vi "Demultiplexer_Laser80VerySimple160.vi"() -> ()   [LabVIEW 2012]
uses:
  <vilib>/Platform/TimedLoop/XDataNode/timing_clust.ctl
  <vilib>/Platform/TimedLoop/XDataNode/nitl_modes.ctl
  <vilib>/Platform/TimedLoop/XDataNode/wakeup.ctl
  <vilib>/rvi/Emulation/niFpgaSctlEmulationRegisterWithScheduler.vi
  <vilib>/rvi/eio/common/nirviEmuTemplateMethod_errors.vi
  <vilib>/rvi/Emulation/niFpgaSctlEmulationScheduler.vi
  <vilib>/rvi/FIFO/Fifo_Resource/nirvififoEmulationSetSize.vi
  <vilib>/rvi/DataTransferAndStorage/Container/Common/niFpgaContainerGetUniqueNameForEmu.vi
  <vilib>/rvi/errors/niFpgaSetErrorForExecOnDevCompSimple.vi
  <vilib>/rvi/eio/common/nirviEmuReportErrorAndStop.vi
  <vilib>/rvi/Emulation/niFpgaSctlEmulationFifoFullMgr.vi
  <vilib>/rvi/Emulation/niFpgaSctlEmulationResourceMgr.vi
  <vilib>/rvi/interface/RandomDataEmulation/nirviRandomDataFPGAFIFO.vi
  <vilib>/rvi/interface/RandomDataEmulation/niFpgaRandomDataHandleErrors.vi
  <vilib>/rvi/Emulation/niFpgaSctlEmulationGlobalWrite.vi
  <vilib>/Platform/TimedLoop/XDataNode/XDataNode.xnode
  <vilib>/eio/EIONode/EIONode.xnode
  <vilib>/rvi/DataTransferAndStorage/Container/XNode/niFpgaContainer.xnode
  <vilib>/rvi/FIFO/Fifo_Resource/nirvififoEmulationClear.vi
  <vilib>/rvi/FIFO/Fifo_Resource/nirvififoEmulationWrite.vi
  <vilib>/rvi/FIFO/Fifo_Resource/nirvififoEmulationRead.vi
  <vilib>/rvi/interface/RandomDataEmulation/nirviRandomDataFpgaReadWriteTemplate.vi
  <vilib>/Platform/TimedLoop/XDataNode/XDNodeRunTimeDep.lvlib
panel:
  out "Laser pulses per pixel A1":u16
  out "ToHost FIFO Overflow A2Ch2":bool
  out "ToHost FIFO Overflow A2Ch1":bool
  out "ToHost FIFO Overflow A1Ch2":bool
  in  "Samples per pixel Acq A2":u16=10000 caption="Samples per pixel Acq"
  in  "Samples per pixel Acq A1":u16=10000 caption="Samples per pixel Acq"
  in  "Requested pixels A2":u32=100000 caption="Requested pixels"
  in  "Samples per pixel A2":u16=10000 caption="Samples per pixel"
  out "ToHost FIFO Overflow A1Ch1":bool
  out "Acquiring":bool
  in  "Wait for trigger":bool
  in  "Acquire continuously":bool=TRUE
  in  "Requested pixels A1":u32=100000 caption="Requested pixels"
  in  "Clear Interloop FIFO":bool
  out "Interloop FIFO overflow":bool
  in  "Samples per pixel A1":u16=10000 caption="Samples per pixel"
  in  "Acquire":bool
  out "Interloop FIFO timeout":bool
  in  "Commit":bool
  out "Xpoint_Switch_Ready":bool
  in  "Xpoint_Switch_Write":bool
  in  "Clock Source":u8(ring)=3 items=["Tristate"=0, "Sync Clock (PXIe only)"=2, "Adapter Module Onboard Clock"=3, "Strobe from Crosspoint Switch"=4, "Strobe Bypass"=5]
  in  "Onboard_Clock_Write":bool
  in  "Onboard_Clock_Write_Data":u16
  out "Onboard_Clock_Ready":bool
  in  "Acq_Reset":bool
  # "6587 IO module configuration"
  # "Demultiplexer - Laser 80MHzVerySimple160MHz"
  # "Acquisition control"
  # "Area 1"
  # "Area 2"
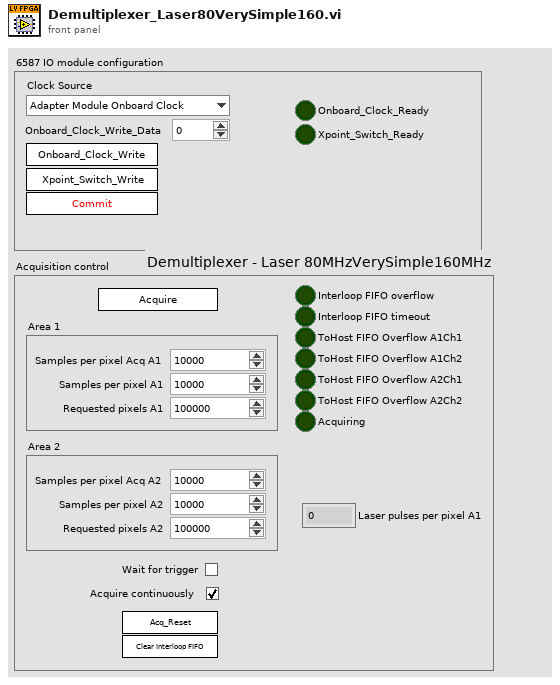
[diagram p1: front panel]
types:
  T1 = typedef "XDNodeRunTimeDep.lvlib/timing_clust.ctl" = cluster{"Expected End [f-1]":u64, "Actual End [f-1]":u64, "Finished Late? [f-1]":bool, "Expected End [i-1]":u64, "Actual End [i-1]":u64, "Finished Late? [i-1]":bool, "Expected Start [i]":u64, "Actual Start [i]":u64, "Expected Start [f]":u64, "Actual Start [f]":u64, "Source Name":string, "Structure Name":string, "Period":i64, "Deadline":i64, "Offset":i64, "Start":i64, "Priority":i32, "Timeout":i32, "Mode":T2, "Wakeup Reason":T3, "Error":errorcluster, "Source Type":string, "Secondary Source Type":string, "Global End Time":u64, "Global Start Time":u64, "Frame Duration":u64, "Iteration Duration":u64, "Assigned CPU":i32, "I/O Scan Engine Mode":u32}
  T2 = typedef "XDNodeRunTimeDep.lvlib/nitl_modes.ctl" = enum32{"No Change", "Process missed periods, maintain original phase", "Discard missed periods, maintain original phase", "Process missed periods, ignore original phase", "Discard missed periods, ignore original phase"}
  T3 = typedef "XDNodeRunTimeDep.lvlib/wakeup.ctl" = enum32{"Normal", "Aborted", "Asynchronous wakeup", "Timing source error", "Timed loop error", "Timeout"}
  T4 = cluster{"Laser":u64, "A1Ch1":u64, "A1Ch2":u64, "A2Ch1":u64, "A2Ch2":u64}
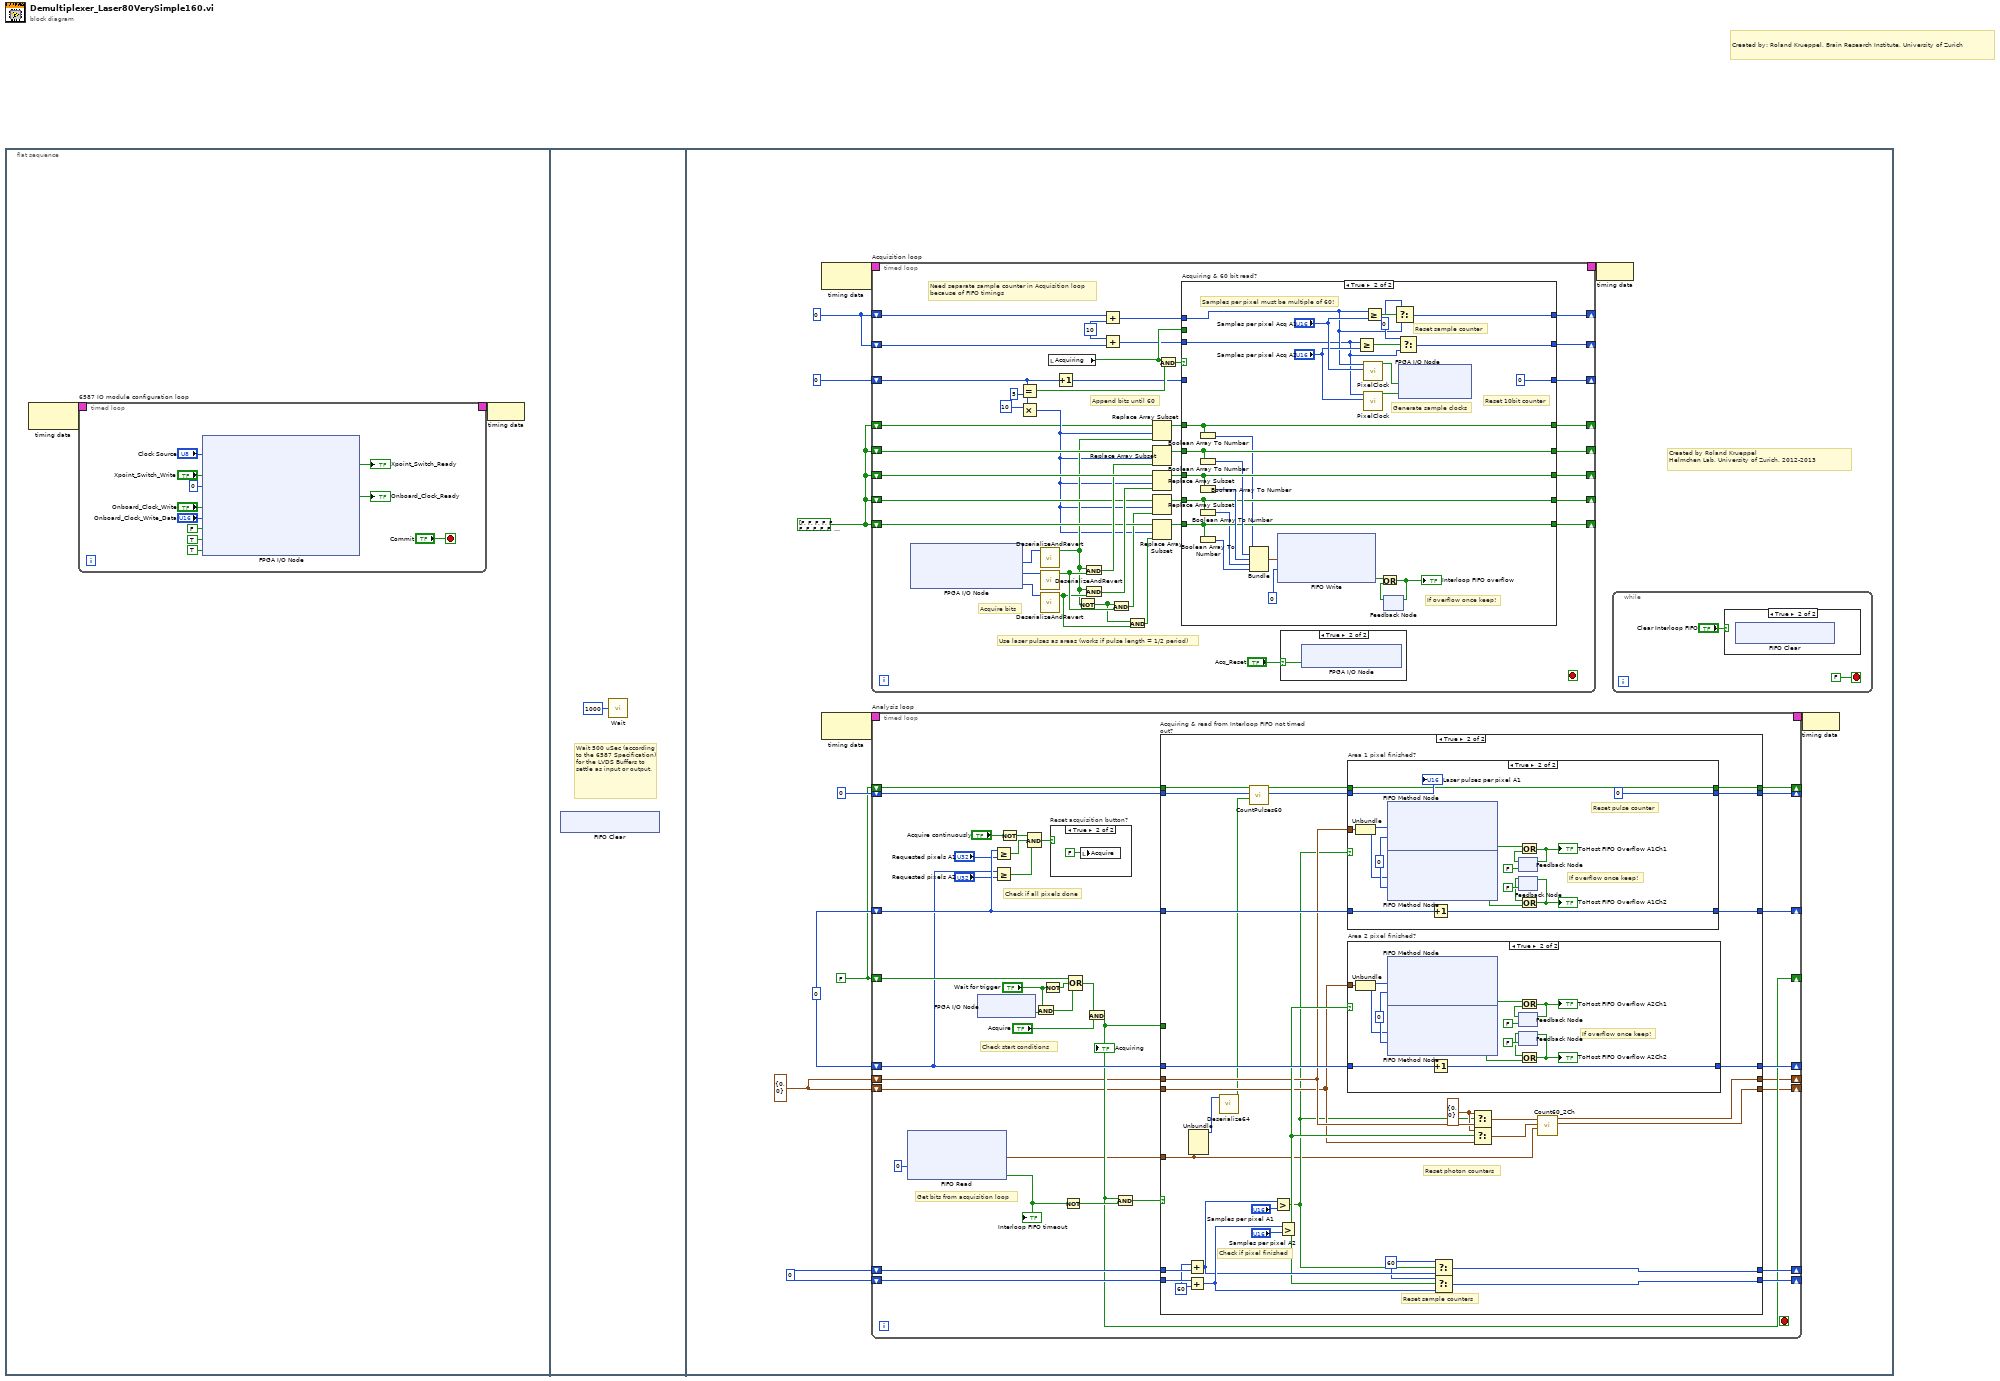
[diagram p0: block diagram]
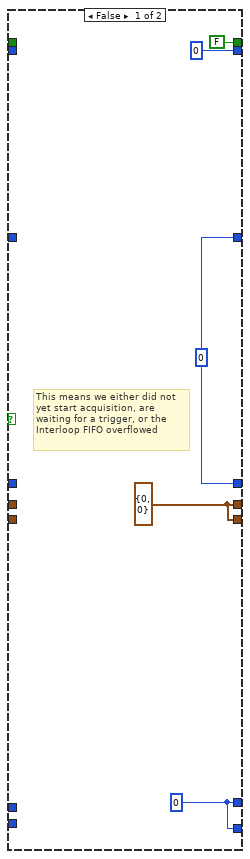
[diagram p5: hidden frame]
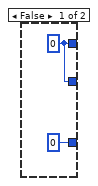
[diagram p10: hidden frame]
diagram:
  # "Created by: Roland Krueppel, Brain Research Institute, University of Zurich"
  n1 = flat-sequence {
    frame #0 {
      n2 = node-c288() -> (w2:T1)  [unwired: 1 in]
      n3 = timed-loop "6587 IO module configuration loop" {
        timing: w2 -> [_]
        timing-out: [_] -> w1
        stop <- "Commit" stop-if-true
        n4 = xnode "FPGA I/O Node"("IO Module\\Acq_IO_Clock_Source"="Clock Source", "IO Module\\Xpoint_Switch_Write"="Xpoint_Switch_Write", "IO Module\\LVDS_Data_Dir"=u16 0 ("IO Module\\LVDS_Data_Dir"), "IO Module\\Onboard_Clock_Write"="Onboard_Clock_Write", "IO Module\\Onboard_Clock_Write_Data"="Onboard_Clock_Write_Data", "IO Module\\SE_PFI0_WE"=FALSE ("IO Module\\SE_PFI0_WE"), "IO Module\\SE_PFI1_WE"=TRUE ("IO Module\\SE_PFI1_WE"), "IO Module\\SE_PFI2_WE"=TRUE ("IO Module\\SE_PFI2_WE")) -> ("IO Module\\Xpoint_Switch_Ready"=→"Xpoint_Switch_Ready":bool, "IO Module\\Onboard_Clock_Ready"=→"Onboard_Clock_Ready":bool)  [unwired: 10 in, 10 out]
      }
      n5 = node-c288(w1) -> ()
    }
    frame #1 {
      # "Wait 500 uSec (according to the 6587 Specification) for the LVDS Buffers to settle as input or output."
      n6 = xnode ("FIFO Clear")() -> ()  [unwired: 1 in, 1 out]
      n7 = call "Wait"("Count(uSec)"=u32 1000) -> ()  [unwired: 1 out]
    }
    frame #2 {
      w23 = cluster{u16, u16} {0, 0} ("output cluster")
      w24 = u16 0
      w22 = u32 0 ("Cycle counter out")
      w25 = u16 0
      w21 = bool[] [FALSE, FALSE, FALSE, FALSE, FALSE, FALSE, FALSE, FALSE, FALSE, FALSE, FALSE, FALSE, FALSE, FALSE, FALSE, FALSE, FALSE, FALSE, FALSE, FALSE, FALSE, FALSE, FALSE, FALSE, FALSE, FALSE, FALSE, FALSE, FALSE, FALSE, FALSE, FALSE, FALSE, FALSE, FALSE, FALSE, FALSE, FALSE, FALSE, FALSE, FALSE, FALSE, FALSE, FALSE, FALSE, FALSE, FALSE, FALSE, FALSE, FALSE, FALSE, FALSE, FALSE, FALSE, FALSE, FALSE, FALSE, FALSE, FALSE, FALSE, FALSE, FALSE, FALSE, FALSE] ("Boolean array")
      w19 = FALSE ("Last laser bit out")
      # "Created by Roland Krueppel\nHelmchen Lab, University of Zurich, 2012-2013"
      n8 = node-c288() -> (w30:T1)  [unwired: 1 in]
      n9 = node-c288() -> (w28:T1)  [unwired: 1 in]
      n10 = timed-loop "Acquisition loop" {
        timing: w30 -> [_]
        timing-out: [_] -> w29
        shift-right: [w207] -> _
        shift-left: w21 -> [w213]
        shift-right: [w206] -> _
        shift-left: 0 -> [w205]
        shift-right: [w202] -> _
        shift-left: w21 -> [w204]
        shift-right: [w201] -> _
        shift-left: w24 -> [w194]
        shift-right: [w200] -> _
        shift-left: w24 -> [w192]
        shift-right: [w177] -> _
        shift-left: w21 -> [w186]
        shift-right: [w176] -> _
        shift-left: w21 -> [w185]
        shift-right: [w171] -> _
        shift-left: w21 -> [w173]
        stop <- _ stop-if-true
        w190 = u16 10 ("y")
        # "Use laser pulses as areas (works if pulse length = 1/2 period)"
        # "Need separate sample counter in Acquisition loop\nbecause of FIFO timings"
        # "Append bits until 60"
        # "Acquire bits"
        n11 = xnode "FPGA I/O Node"() -> ("IO Module\\LVDS_Ch0_Rd"=w197:u16, "IO Module\\LVDS_Ch1_Rd"=w196:u16, "IO Module\\LVDS_Ch2_Rd"=w195:u16)  [unwired: 3 in, 3 out]
        n12 = Equal?(x=w205, y=5) -> (x = y?=w210:bool)
        n13 = Multiply(x=10 ("y"), y=w205) -> (x*y=w174:i32)
        n14 = call "DeserializeAndRevert.vi"("U16 input"=w197) -> ("10bit output"=w175:bool[])  [unwired: 10 in]
        n15 = call "DeserializeAndRevert.vi"("U16 input"=w196) -> ("10bit output"=w184:bool[])  [unwired: 10 in]
        n16 = call "DeserializeAndRevert.vi"("U16 input"=w195) -> ("10bit output"=w182:bool[])  [unwired: 10 in]
        n17 = local read "Acquiring"() -> (w199:bool)
        n18 = Increment(x=w205) -> (x+1=w198:i32)
        n19 = Not(x=w175) -> (.not. x?=w183:bool[])
        n20 = And(x=w175, y=w184) -> (x .and. y?=w187:bool[])
        n21 = And(x=w175, y=w182) -> (x .and. y?=w188:bool[])
        n22 = Add(x=w194, y=w190) -> (x+y=w193:u16)
        n23 = Add(x=w190, y=w192) -> (x+y=w191:u16)
        n24 = And(x=w183, y=w184) -> (x .and. y?=w181:bool[])
        n25 = And(x=w183, y=w182) -> (x .and. y?=w180:bool[])
        n26 = Replace Array Subset(array=w173, new element=w175, index=w174) -> (w172:bool[])
        n27 = Replace Array Subset(array=w213, new element=w187, index=w174) -> (w208:bool[])
        n28 = Replace Array Subset(array=w204, new element=w188, index=w174) -> (w203:bool[])
        n29 = Replace Array Subset(array=w186, new element=w181, index=w174) -> (w179:bool[])
        n30 = Replace Array Subset(array=w185, new element=w180, index=w174) -> (w178:bool[])
        n31 = And(x=w199, y=w210) -> (x .and. y?=w209:bool)
        n32 = case "Acquiring & 60 bit read?" shown="True" w209 {
          tunnel: w208 -> [w226 w257]
          tunnel: [w226 w257] -> w207
          tunnel: [w218 0] -> w206
          tunnel: w198 -> [w219 _]
          tunnel: w203 -> [w225 w256]
          tunnel: [w225 w256] -> w202
          tunnel: w193 -> [w223 w245]
          tunnel: [w220 w254] -> w201
          tunnel: w191 -> [w222 w244]
          tunnel: [w221 w249] -> w200
          tunnel: w199 -> [w224 _]
          tunnel: w179 -> [w217 w238]
          tunnel: w178 -> [w216 w237]
          tunnel: [w217 w238] -> w177
          tunnel: [w216 w237] -> w176
          tunnel: w172 -> [w215 w233]
          tunnel: [w215 w233] -> w171
          frame False {
            n33 = case "Acquiring?" shown="True" w224 {
              tunnel: w223 -> [_ w231]
              tunnel: w222 -> [_ w230]
              tunnel: [w228 w231] -> w220
              tunnel: [w228 w230] -> w221
              tunnel: w219 -> [_ w229]
              tunnel: [0 w229] -> w218
              frame False {
                w228 = u16 0
              }
              frame True {
              }
            }
          }
          frame True {
            w250 = u16 0 ("t")
            # "Reset 10bit counter"
            # "Samples per pixel must be multiple of 60!"
            # "Reset sample counter"
            # "If overflow once keep!"
            # "Generate sample clocks"
            n34 = Boolean Array To Number(Boolean array=w233) -> (number=w232:u64)
            n35 = Boolean Array To Number(Boolean array=w257) -> (number=w240:u64)
            n36 = Boolean Array To Number(Boolean array=w256) -> (number=w239:u64)
            n37 = Boolean Array To Number(Boolean array=w238) -> (number=w236:u64)
            n38 = Boolean Array To Number(Boolean array=w237) -> (number=w235:u64)
            n39 = Bundle(w232, w240, w239, w236, w235) -> (w234:cluster{u64, u64, u64, u64, u64})  [unwired: 1 in]
            n40 = xnode ("FIFO Write")("Element"=w234, "Timeout"=0) -> ("Timed Out?"=w243:bool)  [unwired: 1 in, 1 out]
            n41 = Greater Or Equal?(x=w244, y="Samples per pixel Acq A2") -> (x >= y?=w251:bool)
            n42 = call "PixelClock.vi"("Samples per pixel"="Samples per pixel Acq A1", "Sample counter"=w245) -> ("Pixel clock"=w252:bool)  [unwired: 9 in]
            n43 = call "PixelClock.vi"("Samples per pixel"="Samples per pixel Acq A2", "Sample counter"=w244) -> ("Pixel clock"=w247:bool)  [unwired: 9 in]
            n44 = Greater Or Equal?(x=w245, y="Samples per pixel Acq A1") -> (x >= y?=w255:bool)
            n45 = feedback #1() -> (w241:bool)  [unwired: 1 in]
            n46 = Or(x=w243, y=w241) -> (x .or. y?=w242:bool)
            "Interloop FIFO overflow" <- w242
            n47 = feedback-in #1(w242) -> ()
            n48 = Select(t=w250, s=w255, f=w245) -> (s? t:f=w254:u16)
            n49 = Select(t=w250, s=w251, f=w244) -> (s? t:f=w249:u16)
            n50 = xnode "FPGA I/O Node"("Pixel clock A1"=w252, "Pixel clock A2"=w247) -> ()  [unwired: 2 in, 2 out]
          }
        }
        n51 = case shown="True" "Acq_Reset" {
          selector: "Acq_Reset" -> [_ w214]
          frame False {
          }
          frame True {
            n52 = xnode "FPGA I/O Node"("IO Module\\Acq_Reset"=w214) -> ()  [unwired: 1 in, 1 out]
          }
        }
      }
      n53 = timed-loop "Analysis loop" {
        timing: w28 -> [_]
        timing-out: [_] -> w27
        shift-right: [w48] -> _
        shift-left: w25 -> [w68]
        shift-right: [w46] -> _
        shift-left: w22 -> [w67]
        shift-right: [w44] -> _
        shift-left: w19 -> [w56]
        shift-right: [w47] -> _
        shift-left: w25 -> [w54]
        shift-right: [w45] -> _
        shift-left: w22 -> [w52]
        shift-right: [w39] -> _
        shift-left: w23 -> [w41]
        shift-right: [w38] -> _
        shift-left: w23 -> [w40]
        shift-right: [w36] -> _
        shift-left: u16 0 ("New pulse count") -> [w35]
        shift-right: [w34] -> _
        shift-left: w19 -> [w33]
        stop <- _ stop-if-true
        # "Get bits from acquisition loop"
        # "Check start conditions"
        # "Check if all pixels done"
        n54 = xnode ("FIFO Read")("Timeout"=0) -> ("Element"=w37:T4, "Timed Out?"=w42:bool)  [unwired: 1 in, 1 out]
        "Interloop FIFO timeout" <- w42
        n55 = xnode "FPGA I/O Node"() -> ("TriggerIn"=w62:bool)  [unwired: 1 in, 1 out]
        n56 = Greater Or Equal?(x=w67, y="Requested pixels A1") -> (x >= y?=w50:bool)
        n57 = Greater Or Equal?(x=w52, y="Requested pixels A2") -> (x >= y?=w49:bool)
        n58 = Not(x="Acquire continuously") -> (.not. x?=w51:bool)
        n59 = Compound Arithmetic op=AND(w51, w50, w49) -> (w64:bool)
        n60 = And(x="Wait for trigger", y=w62) -> (x .and. y?=w59:bool)
        n61 = Not(x="Wait for trigger") -> (.not. x?=w60:bool)
        n62 = case "Reset acquisition button?" shown="True" w64 {
          frame False {
          }
          frame True {
            n63 = local write "Acquire"(FALSE ("Acquire")) -> ()
          }
        }
        n64 = Not(x=w42) -> (.not. x?=w57:bool)
        n65 = Compound Arithmetic op=OR(w56, w60, w59) -> (w58:bool)
        n66 = And(x=w58, y="Acquire") -> (x .and. y?=w44:bool)
        "Acquiring" <- w44
        n67 = And(x=w44, y=w57) -> (x .and. y?=w55:bool)
        n68 = case "Acquiring & read from Interloop FIFO not timed out?" shown="True" w55 {
          tunnel: w41 -> [w85 w116]
          tunnel: w68 -> [w84 w131]
          tunnel: w67 -> [w83 w127]
          tunnel: w44 -> [w86 _]
          tunnel: w54 -> [w77 w129]
          tunnel: w52 -> [w80 w126]
          tunnel: [w78 w119] -> w48
          tunnel: [w76 w121] -> w47
          tunnel: [w82 w110] -> w39
          tunnel: [w81 w124] -> w46
          tunnel: [w79 w125] -> w45
          tunnel: w40 -> [w75 w115]
          tunnel: [w74 w109] -> w38
          tunnel: w37 -> [_ w108]
          tunnel: [w70 w103] -> w36
          tunnel: w35 -> [w72 w102]
          tunnel: [w71 w101] -> w34
          tunnel: w33 -> [w73 w100]
          frame False {
            n69 = case "Acquiring?" shown="True" w86 {
              tunnel: w85 -> [_ w99]
              tunnel: w84 -> [_ w96]
              tunnel: w83 -> [_ w98]
              tunnel: [w90 w99] -> w82
              tunnel: [w91 w98] -> w81
              tunnel: w80 -> [_ w97]
              tunnel: [w91 w97] -> w79
              tunnel: [w89 w96] -> w78
              tunnel: [w89 w95] -> w76
              tunnel: w77 -> [_ w95]
              tunnel: w75 -> [_ w94]
              tunnel: [w90 w94] -> w74
              tunnel: w73 -> [_ w93]
              tunnel: w72 -> [_ w92]
              tunnel: [FALSE ("Last laser bit out") w93] -> w71
              tunnel: [u16 0 ("New pulse count") w92] -> w70
              frame False {
                w90 = cluster{u16, u16} {0, 0} ("output cluster")
                w91 = u32 0 ("Cycle counter out")
                w89 = u16 0
                # "This means we either did not\nyet start acquisition, are\nwaiting for a trigger, or the\nInterloop FIFO overflowed"
              }
              frame True {
                # "This means we are\nreading faster here\nthan acquiring in\nAcquisition loop\n-> keep all values"
              }
            }
          }
          frame True {
            w114 = cluster{u16, u16} {0, 0} ("t")
            w118 = u16 60 ("t")
            w128 = u16 60
            # "Reset photon counters"
            # "Check if pixel finished"
            # "Reset sample counters"
            n70 = Add(x=w128, y=w131) -> (x+y=w120:u16)
            n71 = Add(x=w129, y=w128) -> (x+y=w122:u16)
            n72 = Unbundle(w108) -> ("Laser"=w107:u64)  [unwired: 4 out]
            n73 = call "Deserialize64.vi"("U64 input"=w107) -> ("60bit output"=w106:bool[])  [unwired: 10 in]
            n74 = call "CountPulses60.vi"("60bit input"=w106, "Previous pulse count"=w102, "Last sample"=w100) -> ("New pulse count"=w105:u16, "New last sample"=w104:bool)  [unwired: 7 in]
            n75 = Greater?(x=w120, y="Samples per pixel A1") -> (0:w113:bool)
            n76 = Greater?(x=w122, y="Samples per pixel A2") -> (0:w117:bool)
            n77 = case "Area 1 pixel finished?" shown="True" w113 {
              tunnel: w116 -> [_ w163]
              tunnel: w127 -> [w149 w165]
              tunnel: [w149 w164] -> w124
              tunnel: w105 -> [w147 w152]
              tunnel: w104 -> [w148 w151]
              tunnel: [w147 u16 0 ("New pulse count")] -> w103
              tunnel: [w148 w151] -> w101
              frame False {
              }
              frame True {
                w166 = 0 ("Timeout")
                # "Reset pulse counter"
                # "If overflow once keep!"
                n78 = Unbundle(w163) -> (w162:u16, w161:u16)
                n79 = xnode ("FIFO Method Node")("Element"=w162, "Timeout"=w166) -> ("Timed Out?"=w156:bool)  [unwired: 1 in, 1 out]
                n80 = xnode ("FIFO Method Node")("Element"=w161, "Timeout"=w166) -> ("Timed Out?"=w155:bool)  [unwired: 1 in, 1 out]
                n81 = Increment(x=w165) -> (x+1=w164:u32)
                n82 = feedback #2(FALSE) -> (w160:bool)
                n83 = feedback #3(FALSE) -> (w157:bool)
                n84 = Or(x=w156, y=w160) -> (x .or. y?=w154:bool)
                "ToHost FIFO Overflow A1Ch1" <- w154
                n85 = feedback-in #2(w154) -> ()
                n86 = Or(x=w157, y=w155) -> (x .or. y?=w153:bool)
                "ToHost FIFO Overflow A1Ch2" <- w153
                n87 = feedback-in #3(w153) -> ()
                "Laser pulses per pixel A1" <- w152
              }
            }
            n88 = case "Area 2 pixel finished?" shown="True" w117 {
              tunnel: w126 -> [w132 w145]
              tunnel: [w132 w144] -> w125
              tunnel: w115 -> [_ w143]
              frame False {
              }
              frame True {
                w146 = 0 ("Timeout")
                # "If overflow once keep!"
                n89 = Unbundle(w143) -> (w142:u16, w141:u16)
                n90 = xnode ("FIFO Method Node")("Element"=w142, "Timeout"=w146) -> ("Timed Out?"=w136:bool)  [unwired: 1 in, 1 out]
                n91 = xnode ("FIFO Method Node")("Element"=w141, "Timeout"=w146) -> ("Timed Out?"=w135:bool)  [unwired: 1 in, 1 out]
                n92 = Increment(x=w145) -> (x+1=w144:u32)
                n93 = feedback #4(FALSE) -> (w140:bool)
                n94 = feedback #5(FALSE) -> (w137:bool)
                n95 = Or(x=w136, y=w140) -> (x .or. y?=w134:bool)
                "ToHost FIFO Overflow A2Ch1" <- w134
                n96 = feedback-in #4(w134) -> ()
                n97 = Or(x=w137, y=w135) -> (x .or. y?=w133:bool)
                "ToHost FIFO Overflow A2Ch2" <- w133
                n98 = feedback-in #5(w133) -> ()
              }
            }
            n99 = Select(t=w118, s=w113, f=w120) -> (s? t:f=w119:u16)
            n100 = Select(t=w118, s=w117, f=w122) -> (s? t:f=w121:u16)
            n101 = Select(t=w114, s=w113, f=w116) -> (s? t:f=w112:cluster{u16, u16})
            n102 = Select(t=w114, s=w117, f=w115) -> (s? t:f=w111:cluster{u16, u16})
            n103 = call "Count60_2Ch.vi"("Area interloop cluster"=w108, "Photon counters area 2 in"=w111, "Photon counters area 1 in"=w112) -> ("Photon counters area 2 out"=w109:cluster{u16, u16}, "Photon counters area 1 out"=w110:cluster{u16, u16})  [unwired: 6 in, 1 out]
          }
        }
      }
      n104 = node-c288(w29) -> ()
      n105 = while {
        stop <- FALSE stop-if-true
        n106 = case shown="True" "Clear Interloop FIFO" {
          frame False {
          }
          frame True {
            n107 = xnode ("FIFO Clear")() -> ()  [unwired: 1 in, 1 out]
          }
        }
      }
      n108 = node-c288(w27) -> ()
    }
  }
